vi "Read TDMS Comments.vi"(8 "error in (no error)":errorcluster, 11 "path":path) -> (0 "error out":errorcluster, 2 "Notes":string, 3 "file path out":path)   [LabVIEW 2016, in "Data.TDMS.lvclass"]
uses:
  Data.TDMS.lvclass
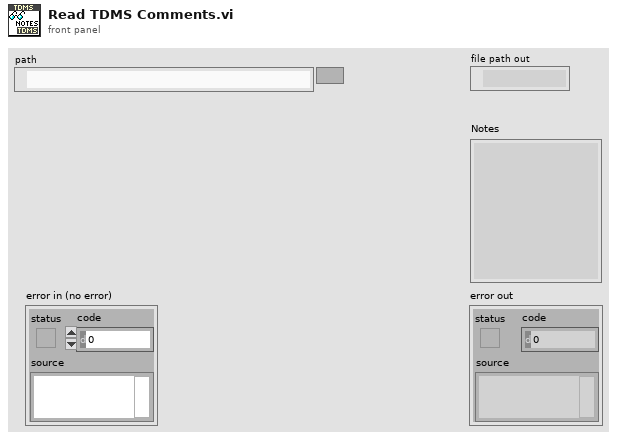
[diagram p1: front panel]
types:
  T1 = enum16{"open", "open or create", "create or replace", "create", "open (read-only)"}
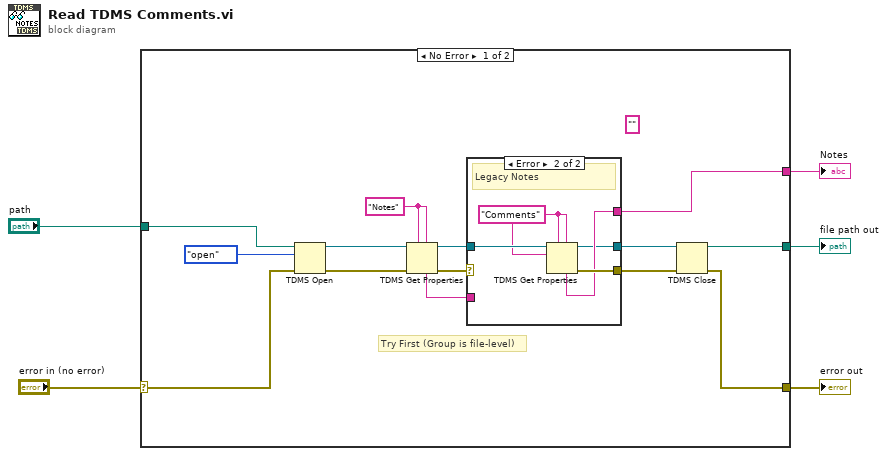
[diagram p0: block diagram]
diagram:
  n1 = case shown="No Error" "error in (no error)" {
    selector: "error in (no error)" -> [w14 w28]
    tunnel: [w16 w28] -> w4
    tunnel: "path" -> [w15 _]
    tunnel: [w8 _] -> w2
    tunnel: [w13 _] -> w1
    frame No Error {
      (unwired) "" ("group name")
      w9 = "Notes" ("group name")
      # "Try First (Group is file-level)"
      n2 = TDMS Open(8:w14, 10:T1."open" ("operation (0:open)"), 11:w15) -> (0:w17:errorcluster, 3:w18:refnum<k34>)  [unwired: 4 in]
      n3 = TDMS Get Properties(5:w9, 7:w9, 8:w17, 11:w18) -> (0:w12:errorcluster, 3:w7:refnum<k34>, 4:w11:string)  [unwired: 2 in, 3 out]
      n4 = case shown="Error" w12 {
        selector: w12 -> [w22 _]
        tunnel: [w22 w27] -> w10
        tunnel: w11 -> [w21 _]
        tunnel: [w21 w26] -> w8
        tunnel: w7 -> [w20 w25]
        tunnel: [w20 w24] -> w6
        frame No Error {
        }
        frame Error {
          w23 = "Comments" ("group name")
          # "Legacy Notes"
          n5 = TDMS Get Properties(5:w23, 7:w23, 10:w23, 11:w25) -> (0:w27:errorcluster, 3:w24:refnum<k34>, 4:w26:string)  [unwired: 2 in, 3 out]
        }
      }
      n6 = TDMS Close(8:w10, 11:w6) -> (0:w16:errorcluster, 3:w13:path)
    }
    frame Error {
    }
  }
  "error out" <- w4
  "Notes" <- w2
  "file path out" <- w1
